vi "async metadata channel.vi"(8 "error in (no error)":errorcluster, 10 "channel_out":u64, 11 "h":u64) -> (0 "error out":errorcluster, 1 "function return":u32(ring), 2 "channel_out out":u64, 3 "h out":u64)   [LabVIEW 2023, in "uhd.lvlib"]
doc: "UHD_API uhd_error uhd_async_metadata_channel(\n uhd_async_metadata_handle h, size_t* channel_out);"
uses:
  <userlib>/uhd/uhd.lvlib
  <userlib>/uhd/uhd.dll
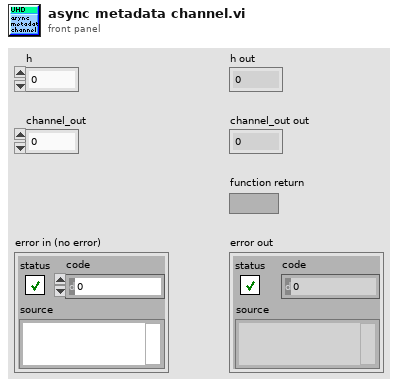
[diagram p1: front panel]
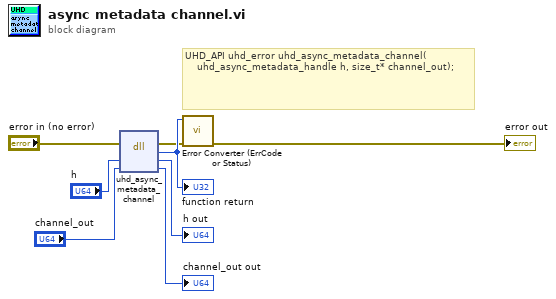
[diagram p0: block diagram]
diagram:
  # "UHD_API uhd_error uhd_async_metadata_channel(\n    uhd_async_metadata_handle h, size_t* channel_out);"
  n1 = dll-call lib="C:/Program Files/National Instruments/LabVIEW 2023/user.lib/uhd/uhd.*" fn="uhd_async_metadata_channel"(error in="error in (no error)", "h"="h", "channel_out"="channel_out") -> (error out=w2:errorcluster, w8:u32, "h"=→"h out":u64, "channel_out"=→"channel_out out":u64)  [unwired: 2 in, 1 out]
  "function return" <- w8
  n2 = call <userlib>:"Error Converter (ErrCode or Status).vi"("error in (no error)"=w2, "error code"=w8) -> ("error out"=→"error out":errorcluster)  [unwired: 9 in]
